vi "Set Offset.vi"(8 "error in (no error)":errorcluster, 11 "IMD in":refnum<class "IMD.lvclass">) -> (0 "error out":errorcluster, 1 "Parameter":cluster{"Name":string, "Value":string}, 2 "Last Offset?":bool, 3 "IMD out":refnum<class "IMD.lvclass">)   [LabVIEW 2020, in "IMD.lvclass"]
uses:
  IMD.lvclass
  IMD.lvclass/IMD.ctl
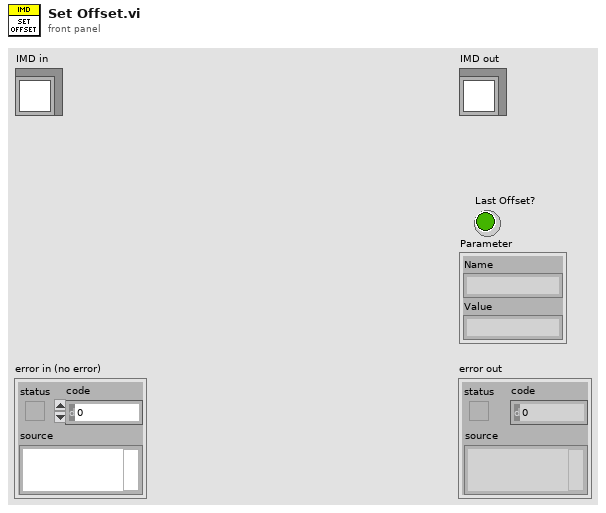
[diagram p1: front panel]
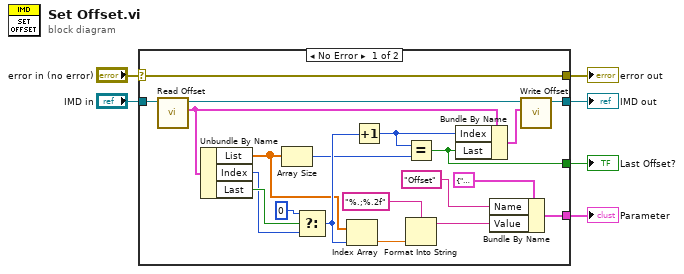
[diagram p0: block diagram]
diagram:
  n1 = case shown="No Error" "error in (no error)" {
    selector: "error in (no error)" -> [w9 w28]
    tunnel: [w9 w28] -> w5
    tunnel: [w10 w27] -> w3
    tunnel: "IMD in" -> [w21 w27]
    tunnel: [w22 _] -> w2
    tunnel: [w12 _] -> w1
    frame No Error {
      n2 = call "Read Offset.vi"("IMD in"=w21) -> ("Offset"=w17:cluster{"List":dbl[], "Index":i32, "Last":bool}, "IMD out"=w20:refnum<class "IMD.lvclass">)  [unwired: 9 in]
      n3 = Unbundle By Name(w17) -> ("List"=w8:dbl[], "Index"=w16:i32, "Last"=w19:bool)
      n4 = Array Size(array=w8) -> (size(s)=w7:i32)
      n5 = Select(t=0, s=w19, f=w16) -> (s? t:f=w15:i32)
      n6 = Index Array(array=w8, index=w15) -> (element=w11:dbl)
      n7 = Increment(x=w15) -> (x+1=w13:i32)
      n8 = Equal?(x=w13, y=w7) -> (x = y?=w12:bool)
      n9 = Format Into String(format string="%.;%.2f", w11) -> (resulting string=w23:string)  [unwired: 2 in, 1 out]
      n10 = Bundle By Name(cluster=w17, "Index"=w13, "Last"=w12) -> (w14:cluster{"List":dbl[], "Index":i32, "Last":bool})
      n11 = Bundle By Name(cluster=cluster{"Name":string, "Value":string} {"Name"="", "Value"=""} ("Change"), "Name"="Offset", "Value"=w23) -> (w22:cluster{"Name":string, "Value":string})
      n12 = call "Write Offset.vi"("Offset"=w14, "IMD in"=w20) -> ("IMD out"=w10:refnum<class "IMD.lvclass">)  [unwired: 9 in]
    }
    frame Error {
    }
  }
  "error out" <- w5
  "IMD out" <- w3
  "Last Offset?" <- w1
  "Parameter" <- w2
